vi "power supply.vi"(7 "Enable Output (T: Enable)":bool=TRUE, 8 "Error In":errorcluster, 10 "Voltage Level (0.0 V)":dbl format="%.3g", 11 "power supply":T1) -> (0 "Error Out":errorcluster)   [LabVIEW 2018]
uses:
  controls/power supply.ctl
  <instrlib>/BK Precision 911X Series/BK Precision 911X Series.lvlib
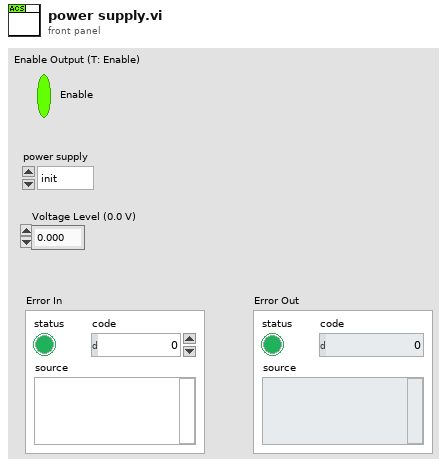
[diagram p1: front panel]
types:
  T1 = typedef "power supply.ctl" = enum16{"init", "set V", "enable", "close"}
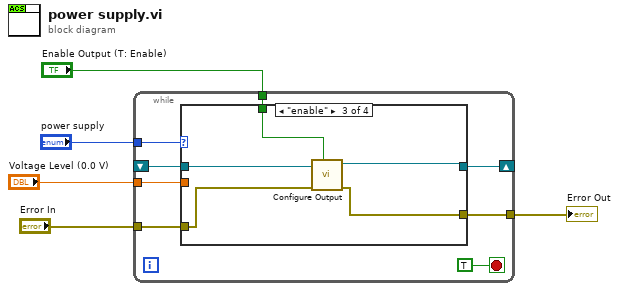
[diagram p0: block diagram]
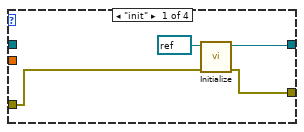
[diagram p2: hidden frame]
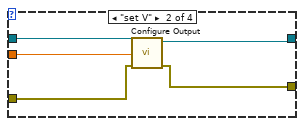
[diagram p3: hidden frame]
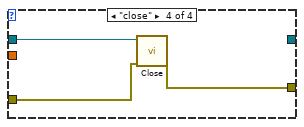
[diagram p4: hidden frame]
diagram:
  n1 = while {
    tunnel: "power supply" -> [w13]
    shift-right: [w12] -> _
    shift-left: _ -> [w10]
    tunnel: "Voltage Level (0.0 V)" -> [w9]
    tunnel: "Enable Output (T: Enable)" -> [w8]
    tunnel: "Error In" -> [w7]
    tunnel: [w6] -> w1
    stop <- TRUE stop-if-true
    n2 = case shown="\"enable\"" w13 {
      tunnel: [w16 w21 w26 _] -> w12
      tunnel: w10 -> [_ w22 w27 w30]
      tunnel: w9 -> [_ w20 _ _]
      tunnel: w8 -> [_ _ w25 _]
      tunnel: w7 -> [w15 w19 w24 w29]
      tunnel: [w14 w18 w23 w28] -> w6
      frame "init" {
        n3 = call <instrlib>:"Initialize.vi"("error in (no error)"=w15, "VISA resource name"=refnum<visa-resource-name> refnum) -> ("error out"=w14:errorcluster, "VISA resource name out"=w16:refnum<visa-resource-name>)  [unwired: 8 in]
      }
      frame "set V" {
        n4 = call <instrlib>:"Configure Output.vi"("error in (no error)"=w19, "Voltage Level (0.0 V)"=w20, "VISA resource name"=w22) -> ("error out"=w18:errorcluster, "VISA resource name out"=w21:refnum<visa-resource-name>)  [unwired: 7 in]
      }
      frame "enable" {
        n5 = call <instrlib>:"Configure Output.vi"("Enable Output (T: Enable)"=w25, "error in (no error)"=w24, "VISA resource name"=w27) -> ("error out"=w23:errorcluster, "VISA resource name out"=w26:refnum<visa-resource-name>)  [unwired: 7 in]
      }
      frame "close" {
        n6 = call <instrlib>:"Close.vi"("error in (no error)"=w29, "VISA resource name"=w30) -> ("error out"=w28:errorcluster)  [unwired: 9 in]
      }
    }
  }
  "Error Out" <- w1
